vi "Leer.vi"() -> ()   [LabVIEW 2019]
panel:
  in  "milliseconds to wait":u32=52
  out "Waveform Chart":dbl(graph)
  in  "stop":bool
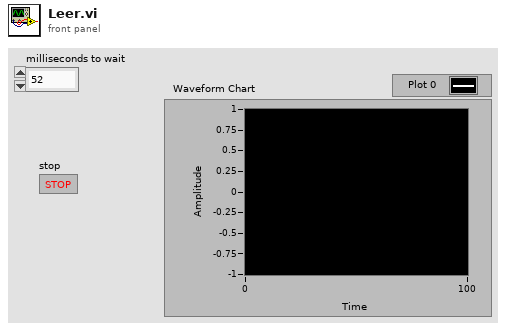
[diagram p1: front panel]
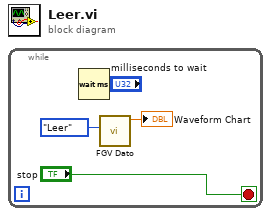
[diagram p0: block diagram]
diagram:
  n1 = while {
    stop <- "stop" stop-if-true
    n2 = Wait (ms)(milliseconds to wait="milliseconds to wait") -> ()  [unwired: 1 out]
    n3 = call "FGV Dato.vi"("Funcion"=enum16{"Guardar", "Leer"}."Leer") -> ("Dato Out"=→"Waveform Chart":dbl)  [unwired: 10 in]
  }
